vi "SurreyRoad_Example_01.vi"() -> ()   [LabVIEW 2010]
panel:
  in  "Set yaw speed":bool
  in  "Start Fans":bool
  in  "stop":bool
  in  "New Percentage":i32
  in  "BL Fan (1 or 2)":i32=1
  out "All Acknowledged?":bool
  in  "EStop":bool
  in  "Stop Yaw":bool
  in  "NewYawPos":dbl
  in  "GotoYaw":bool
  out "YAW POSITION":dbl
  out "?":string
  out "CurrentSpeedSetting":dbl
  in  "NewYawSpeed":dbl
  in  "STOP Road":bool
  in  "Synch to Wind":bool
  in  "GO":bool
  in  "Required_mps":dbl
  out "ROAD SPEED_mps":dbl
  in  "Stop drive":bool
  in  "Start Drive":bool
  out "Road Info":string
  out "Road Status":string
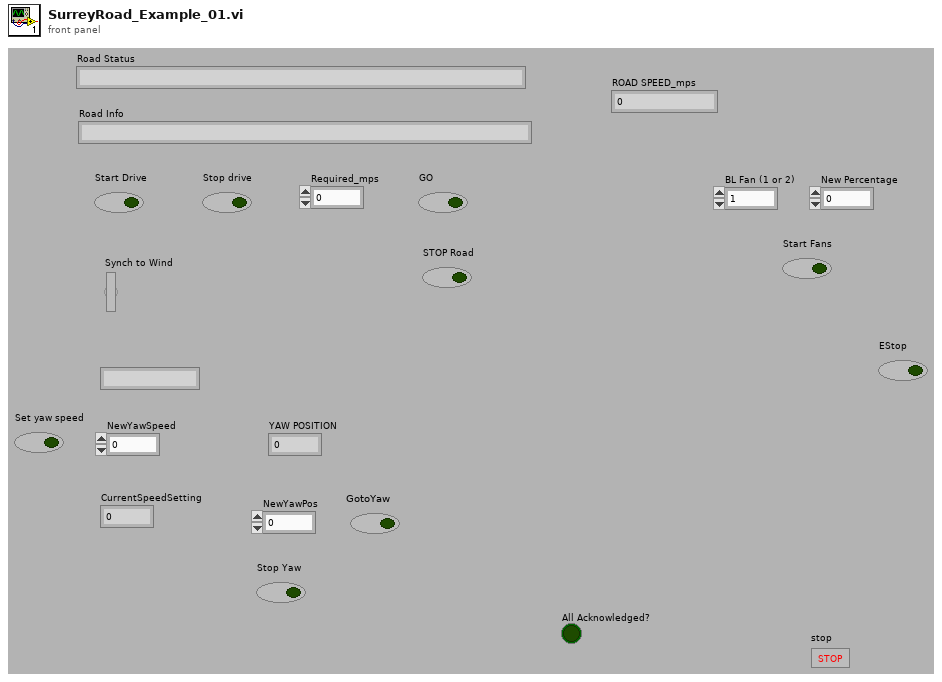
[diagram p1: front panel]
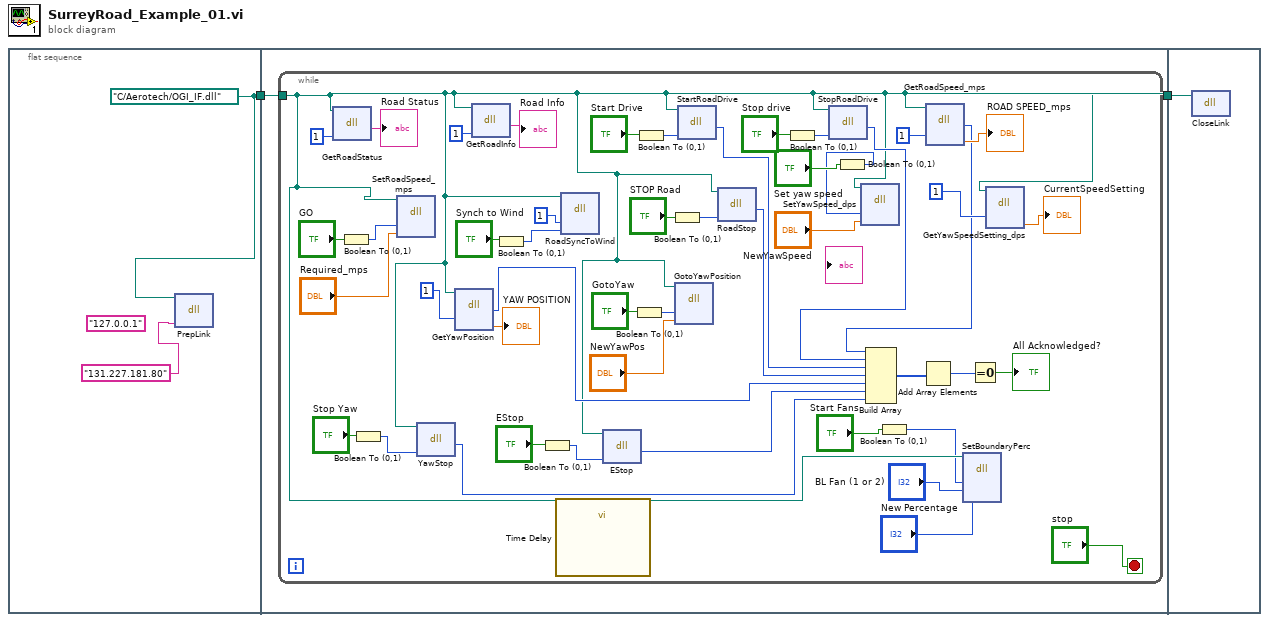
[diagram p0: block diagram]
diagram:
  n1 = flat-sequence {
    tunnel: [w4] -> w2
    tunnel: w2 -> [w5]
    tunnel: [w5] -> w1
    tunnel: w1 -> [w54]
    frame #0 {
      (unwired) "127.0.0.1" ("IPAddress")
      w4 = path "C:/Aerotech/OGI_IF.dll" ("path in")
      n2 = dll-call lib="C:/Aerotech/Drivers/OGI_IF.dll" fn="PrepLink"(path in=w4, "IPAddress"="131.227.181.80") -> ()  [unwired: 2 in, 4 out]
    }
    frame #1 {
      n3 = while {
        tunnel: w5 -> [w14]
        stop <- "stop" stop-if-true
        n4 = dll-call lib="C:/Aerotech/Drivers/OGI_IF.dll" fn="GetRoadStatus"(path in=w14, "Enable"=1) -> ("Road Status"=→"Road Status":string)  [unwired: 3 in, 2 out]
        n5 = Boolean To (0,1)(Boolean="GO") -> (0, 1=w43:i16)
        n6 = Boolean To (0,1)(Boolean="Stop Yaw") -> (0, 1=w30:i16)
        n7 = dll-call lib="C:/Aerotech/Drivers/OGI_IF.dll" fn="SetRoadSpeed_mps"(path in=w14, "Enable"=w43, "Required_mps"="Required_mps") -> ()  [unwired: 3 in, 4 out]
        n8 = dll-call lib="C:/Aerotech/Drivers/OGI_IF.dll" fn="YawStop"(path in=w14, "Enable"=w30) -> ("Acknowledged"=w22:i32)  [unwired: 2 in, 3 out]
        n9 = dll-call lib="C:/Aerotech/Drivers/OGI_IF.dll" fn="GetYawPosition"(path in=w14, "Enable"=1) -> ("Acknowledged"=w24:i32, "Yaw Position"=→"YAW POSITION":dbl)  [unwired: 3 in, 3 out]
        n10 = dll-call lib="C:/Aerotech/Drivers/OGI_IF.dll" fn="GetRoadInfo"(path in=w14, "Enable"=1) -> ("Road Info"=→"Road Info":string)  [unwired: 3 in, 2 out]
        n11 = Boolean To (0,1)(Boolean="Synch to Wind") -> (0, 1=w40:i16)
        n12 = Boolean To (0,1)(Boolean="EStop") -> (0, 1=w28:i16)
        n13 = call "Time Delay"() -> ()  [unwired: 2 in, 10 out]
        n14 = dll-call lib="C:/Aerotech/Drivers/OGI_IF.dll" fn="RoadSyncToWind"(path in=w14, "Enable"=1, "SynchState"=w40) -> ()  [unwired: 3 in, 4 out]
        n15 = dll-call lib="C:/Aerotech/Drivers/OGI_IF.dll" fn="EStop"(path in=w14, "Enable"=w28) -> ("Acknowledged"=w23:i32)  [unwired: 2 in, 3 out]
        n16 = Boolean To (0,1)(Boolean="GotoYaw") -> (0, 1=w33:i16)
        n17 = Boolean To (0,1)(Boolean="Start Drive") -> (0, 1=w50:i16)
        n18 = Boolean To (0,1)(Boolean="STOP Road") -> (0, 1=w39:i16)
        n19 = dll-call lib="C:/Aerotech/Drivers/OGI_IF.dll" fn="GotoYawPosition"(path in=w14, "Enable"=w33, "NewYawPos"="NewYawPos") -> ()  [unwired: 3 in, 4 out]
        n20 = dll-call lib="C:/Aerotech/Drivers/OGI_IF.dll" fn="StartRoadDrive"(path in=w14, "Enable"=w50) -> ("Acknowledged"=w26:i32)  [unwired: 2 in, 3 out]
        n21 = dll-call lib="C:/Aerotech/Drivers/OGI_IF.dll" fn="RoadStop"(path in=w14, "Enable"=w39) -> ("Acknowledged"=w27:i32)  [unwired: 2 in, 3 out]
        n22 = Boolean To (0,1)(Boolean="Stop drive") -> (0, 1=w49:i16)
        n23 = dll-call lib="C:/Aerotech/Drivers/OGI_IF.dll" fn="StopRoadDrive"(path in=w14, "Enable"=w49) -> ("Acknowledged"=w25:i32)  [unwired: 2 in, 3 out]
        n24 = Boolean To (0,1)(Boolean="Set yaw speed") -> (0, 1=w8:i16)
        n25 = dll-call lib="C:/Aerotech/Drivers/OGI_IF.dll" fn="SetYawSpeed_dps"(path in=w14, "Enable"=w8, "NewYawSpeed"="NewYawSpeed") -> ()  [unwired: 3 in, 4 out]
        n26 = Boolean To (0,1)(Boolean="Start Fans") -> (0, 1=w11:i16)
        n27 = dll-call lib="C:/Aerotech/Drivers/OGI_IF.dll" fn="GetRoadSpeed_mps"(path in=w14, "Enable"=1) -> ("Acknowledged"=w13:i32, "RoadSpeed_mps"=→"ROAD SPEED_mps":dbl)  [unwired: 3 in, 3 out]
        n28 = Build Array(w13, w25, w26, w27, w24, w23, w22) -> (w21:i32[])
        n29 = Add Array Elements(numeric array=w21) -> (sum=w18:i32)
        n30 = dll-call lib="C:/Aerotech/Drivers/OGI_IF.dll" fn="SetBoundaryPerc"(path in=w14, "enable"=w11, "BL Fan (1 or 2)"="BL Fan (1 or 2)", "New Percentage"="New Percentage") -> ()  [unwired: 4 in, 4 out]
        n31 = Equal To 0?(x=w18) -> (x = 0?=→"All Acknowledged?":bool)
        n32 = dll-call lib="C:/Aerotech/Drivers/OGI_IF.dll" fn="GetYawSpeedSetting_dps"(path in=w14, "Enable"=1) -> ("CurrentSpeedSetting"=→"CurrentSpeedSetting":dbl)  [unwired: 3 in, 4 out]
      }
    }
    frame #2 {
      n33 = dll-call lib="C:/Aerotech/Drivers/OGI_IF.dll" fn="CloseLink"(path in=w54) -> ()  [unwired: 2 in, 3 out]
    }
  }
